vi "FlushFIFO.vi"(8 "error in (no error)":errorcluster, 11 "9770 API in":refnum<class "9770 API.lvclass">) -> (0 "error out":errorcluster, 3 "9770 API out":refnum<class "9770 API.lvclass">)   [LabVIEW 2017, in "9770 API.lvclass"]
uses:
  <vilib>/addons/InsightCM/Devices/Shared/Emsa/Emsa9770API/9770 API.lvclass
  <vilib>/addons/InsightCM/Devices/Shared/Emsa/Emsa9770API/9770 API.lvclass/9770 API.ctl
  <vilib>/Utility/error.llb/Error Cluster From Error Code.vi
  <vilib>/rvi/errors/niLvFpgaAdjustHostInterfaceError.vi
  <vilib>/rvi/interface/nirviMethod/nirviMethod.xnode
  <vilib>/addons/InsightCM/Devices/Shared/Emsa/Emsa9770API/controls/FPGATypeDef.ctl
  <vilib>/FPGAPlugInAG/Dynamic/niLvFpga_ReadFifo_Dynamic.vi
  <vilib>/rvi/errors/niLvFpgaMergeErrorWithErrorCode.vi
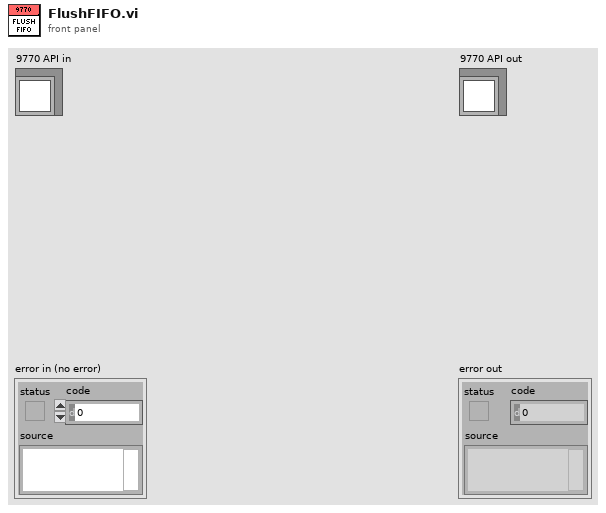
[diagram p1: front panel]
types:
  T1 = typedef "9770 API.lvclass/FPGATypeDef.ctl" = refnum<k20>
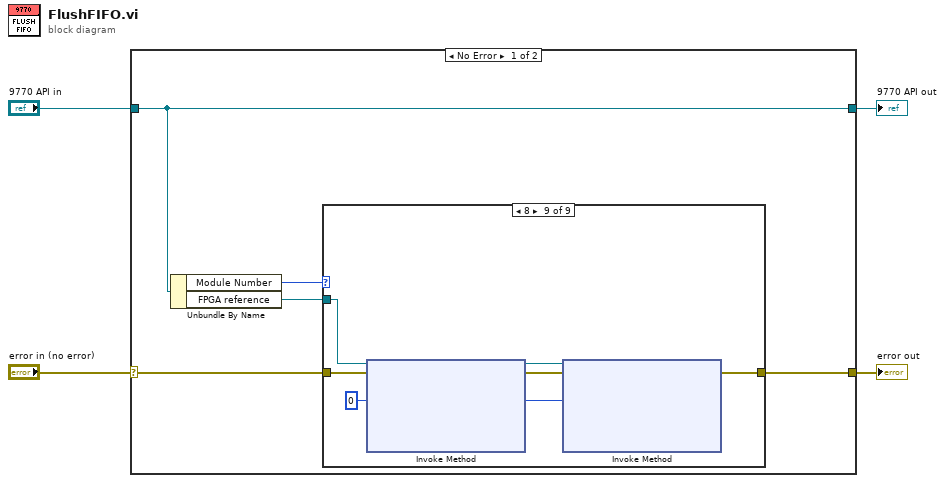
[diagram p0: block diagram]
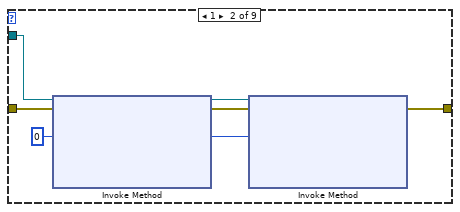
[diagram p3: hidden frame]
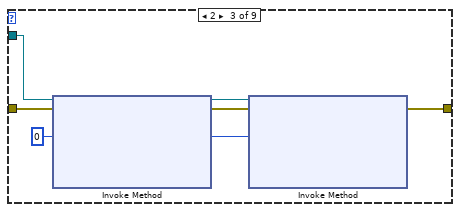
[diagram p4: hidden frame]
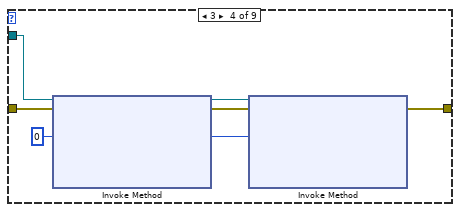
[diagram p5: hidden frame]
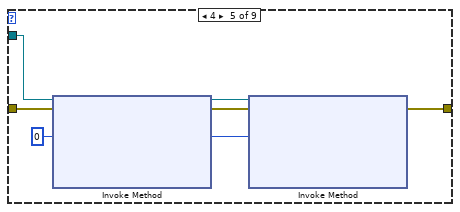
[diagram p6: hidden frame]
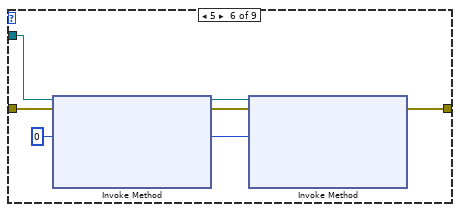
[diagram p7: hidden frame]
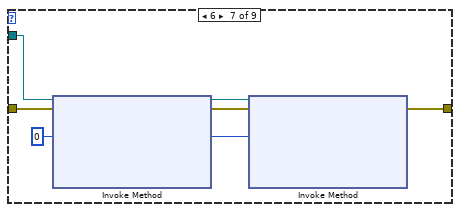
[diagram p8: hidden frame]
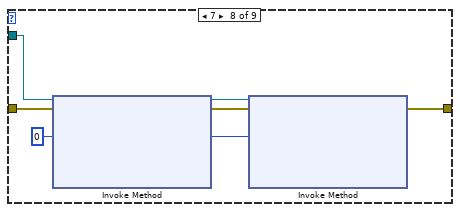
[diagram p9: hidden frame]
diagram:
  n1 = case shown="No Error" "error in (no error)" {
    selector: "error in (no error)" -> [w7 w68]
    tunnel: [w5 w68] -> w3
    tunnel: [w9 w67] -> w1
    tunnel: "9770 API in" -> [w9 w67]
    frame No Error {
      n2 = Unbundle By Name(w9) -> ("Module Number"=w8:u32, "FPGA reference"=w6:T1)
      n3 = case shown="8" w8 {
        tunnel: w7 -> [w10 w13 w20 w27 w34 w41 w48 w55 w62]
        tunnel: w6 -> [_ w12 w19 w26 w33 w40 w47 w54 w61]
        tunnel: [w10 w11 w18 w25 w32 w39 w46 w53 w60] -> w5
        frame 0, Default {
        }
        frame 1 {
          n4 = xnode "Invoke Method"("FPGA VI Reference In"=w12, "error in"=w13, "Number of Elements"=u32 0) -> ("FPGA VI Reference Out"=w16:T1, "error out"=w15:errorcluster, "Elements Remaining"=w14:u32)  [unwired: 1 in, 1 out]
          n5 = xnode "Invoke Method"("FPGA VI Reference In"=w16, "error in"=w15, "Number of Elements"=w14) -> ("error out"=w11:errorcluster)  [unwired: 1 in, 3 out]
        }
        frame 2 {
          n6 = xnode "Invoke Method"("FPGA VI Reference In"=w19, "error in"=w20, "Number of Elements"=u32 0) -> ("FPGA VI Reference Out"=w23:T1, "error out"=w22:errorcluster, "Elements Remaining"=w21:u32)  [unwired: 1 in, 1 out]
          n7 = xnode "Invoke Method"("FPGA VI Reference In"=w23, "error in"=w22, "Number of Elements"=w21) -> ("error out"=w18:errorcluster)  [unwired: 1 in, 3 out]
        }
        frame 3 {
          n8 = xnode "Invoke Method"("FPGA VI Reference In"=w26, "error in"=w27, "Number of Elements"=u32 0) -> ("FPGA VI Reference Out"=w30:T1, "error out"=w29:errorcluster, "Elements Remaining"=w28:u32)  [unwired: 1 in, 1 out]
          n9 = xnode "Invoke Method"("FPGA VI Reference In"=w30, "error in"=w29, "Number of Elements"=w28) -> ("error out"=w25:errorcluster)  [unwired: 1 in, 3 out]
        }
        frame 4 {
          n10 = xnode "Invoke Method"("FPGA VI Reference In"=w33, "error in"=w34, "Number of Elements"=u32 0) -> ("FPGA VI Reference Out"=w37:T1, "error out"=w36:errorcluster, "Elements Remaining"=w35:u32)  [unwired: 1 in, 1 out]
          n11 = xnode "Invoke Method"("FPGA VI Reference In"=w37, "error in"=w36, "Number of Elements"=w35) -> ("error out"=w32:errorcluster)  [unwired: 1 in, 3 out]
        }
        frame 5 {
          n12 = xnode "Invoke Method"("FPGA VI Reference In"=w40, "error in"=w41, "Number of Elements"=u32 0) -> ("FPGA VI Reference Out"=w44:T1, "error out"=w43:errorcluster, "Elements Remaining"=w42:u32)  [unwired: 1 in, 1 out]
          n13 = xnode "Invoke Method"("FPGA VI Reference In"=w44, "error in"=w43, "Number of Elements"=w42) -> ("error out"=w39:errorcluster)  [unwired: 1 in, 3 out]
        }
        frame 6 {
          n14 = xnode "Invoke Method"("FPGA VI Reference In"=w47, "error in"=w48, "Number of Elements"=u32 0) -> ("FPGA VI Reference Out"=w51:T1, "error out"=w50:errorcluster, "Elements Remaining"=w49:u32)  [unwired: 1 in, 1 out]
          n15 = xnode "Invoke Method"("FPGA VI Reference In"=w51, "error in"=w50, "Number of Elements"=w49) -> ("error out"=w46:errorcluster)  [unwired: 1 in, 3 out]
        }
        frame 7 {
          n16 = xnode "Invoke Method"("FPGA VI Reference In"=w54, "error in"=w55, "Number of Elements"=u32 0) -> ("FPGA VI Reference Out"=w58:T1, "error out"=w57:errorcluster, "Elements Remaining"=w56:u32)  [unwired: 1 in, 1 out]
          n17 = xnode "Invoke Method"("FPGA VI Reference In"=w58, "error in"=w57, "Number of Elements"=w56) -> ("error out"=w53:errorcluster)  [unwired: 1 in, 3 out]
        }
        frame 8 {
          n18 = xnode "Invoke Method"("FPGA VI Reference In"=w61, "error in"=w62, "Number of Elements"=u32 0) -> ("FPGA VI Reference Out"=w65:T1, "error out"=w64:errorcluster, "Elements Remaining"=w63:u32)  [unwired: 1 in, 1 out]
          n19 = xnode "Invoke Method"("FPGA VI Reference In"=w65, "error in"=w64, "Number of Elements"=w63) -> ("error out"=w60:errorcluster)  [unwired: 1 in, 3 out]
        }
      }
    }
    frame Error {
    }
  }
  "error out" <- w3
  "9770 API out" <- w1
